vi "File Loader (SubVI).vi"(7 "Filename In":string) -> (0 "Number of Records":i32, 1 "Filename Out":string, 2 "output cluster":T1)   [LabVIEW 2014]
uses:
  <vilib>/Utility/file.llb/Read From Spreadsheet File (DBL).vi
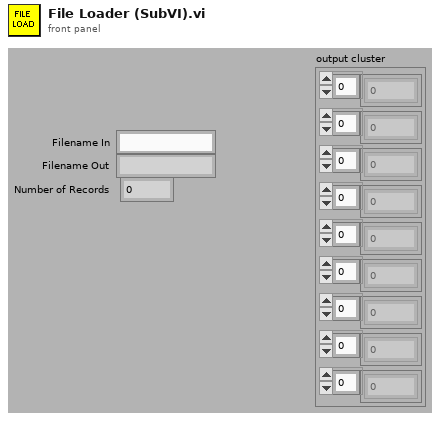
[diagram p1: front panel]
types:
  T1 = cluster{dbl[], dbl[], dbl[], dbl[], dbl[], dbl[], dbl[], dbl[], dbl[]}
  T2 = enum16{"open", "replace", "create", "open or create", "replace or create", "replace or create with confirmation"}
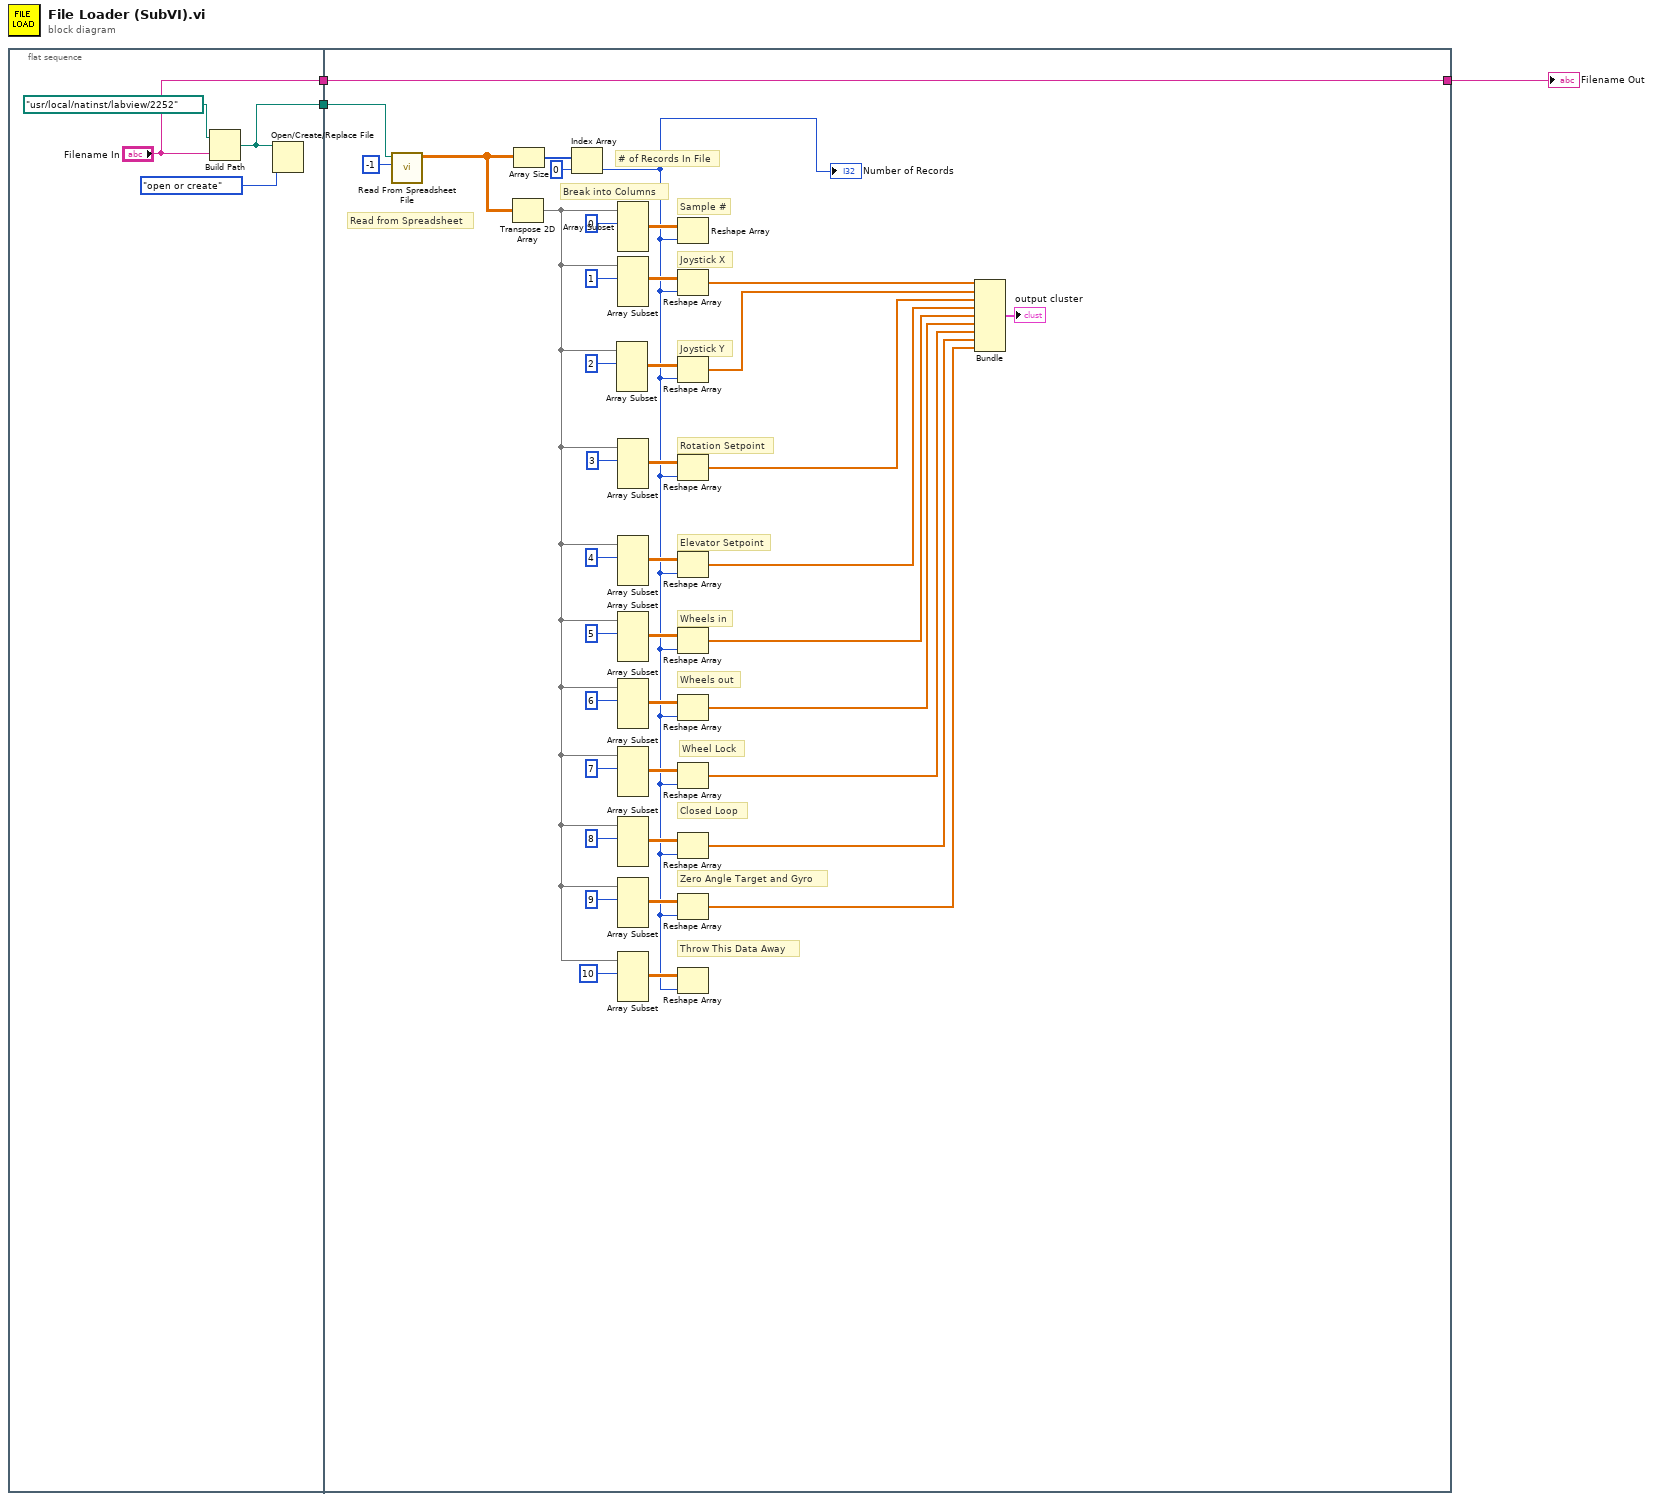
[diagram p0: block diagram]
diagram:
  n1 = flat-sequence {
    tunnel: [w6] -> w3
    tunnel: ["Filename In"] -> w1
    tunnel: w3 -> [w37]
    tunnel: [w34] -> w2
    tunnel: w1 -> [w34]
    frame #0 {
      n2 = Build Path(base path=path "/usr/local/natinst/labview/2252", name or relative path="Filename In") -> (appended path=w6:path)
      n3 = Open/Create/Replace File(file path (use dialog)=w6, operation (0:open)=T2."open or create") -> ()  [unwired: 1 in, 6 out]
    }
    frame #1 {
      # "Wheel Lock"
      # "Throw This Data Away"
      # "Zero Angle Target and Gyro"
      # "Closed Loop"
      # "Wheels out"
      # "Wheels in"
      # "Rotation Setpoint"
      # "Elevator Setpoint"
      # "Break into Columns"
      # "Read from Spreadsheet"
      # "# of Records In File"
      # "Joystick Y"
      # "Joystick X"
      # "Sample #"
      n4 = call-poly <vilib>:"Read From Spreadsheet File.vi"("number of rows (all:-1)"=-1, "file path (dialog if empty)"=w37) -> ("all rows"=w40:dbl[][])  [unwired: 2 in, 7 out]
      n5 = Transpose 2D Array(2D array=w40) -> (transposed array=w10:dbl[][])
      n6 = Array Size(array=w40) -> (size(s)=w39:i32[])
      n7 = Index Array(array=w39, index=0) -> (element=w11:i32)
      "Number of Records" <- w11
      n8 = Array Subset(array=w10, index (row)=2 ("index")) -> (w46:dbl[][])  [unwired: 3 in]
      n9 = Array Subset(array=w10, index (row)=0 ("index")) -> (w44:dbl[][])  [unwired: 3 in]
      n10 = Array Subset(array=w10, index (row)=1 ("index")) -> (w45:dbl[][])  [unwired: 3 in]
      n11 = Array Subset(array=w10, index (row)=3 ("index")) -> (w33:dbl[][])  [unwired: 3 in]
      n12 = Array Subset(array=w10, index (row)=4 ("index")) -> (w35:dbl[][])  [unwired: 3 in]
      n13 = Array Subset(array=w10, index (row)=5 ("index")) -> (w28:dbl[][])  [unwired: 3 in]
      n14 = Array Subset(array=w10, index (row)=6 ("index")) -> (w25:dbl[][])  [unwired: 3 in]
      n15 = Array Subset(array=w10, index (row)=7 ("index")) -> (w24:dbl[][])  [unwired: 3 in]
      n16 = Array Subset(array=w10, index (row)=8 ("index")) -> (w21:dbl[][])  [unwired: 3 in]
      n17 = Array Subset(array=w10, index (row)=9 ("index")) -> (w19:dbl[][])  [unwired: 3 in]
      n18 = Array Subset(array=w10, index (row)=10 ("index")) -> (w13:dbl[][])  [unwired: 3 in]
      n19 = Reshape Array(w44, w11) -> ()  [unwired: 1 out]
      n20 = Reshape Array(w45, w11) -> (w31:dbl[])
      n21 = Reshape Array(w46, w11) -> (w30:dbl[])
      n22 = Reshape Array(w33, w11) -> (w29:dbl[])
      n23 = Reshape Array(w35, w11) -> (w18:dbl[])
      n24 = Reshape Array(w28, w11) -> (w17:dbl[])
      n25 = Reshape Array(w25, w11) -> (w16:dbl[])
      n26 = Reshape Array(w24, w11) -> (w15:dbl[])
      n27 = Reshape Array(w21, w11) -> (w14:dbl[])
      n28 = Reshape Array(w19, w11) -> (w9:dbl[])
      n29 = Reshape Array(w13, w11) -> ()  [unwired: 1 out]
      n30 = Bundle(w31, w30, w29, w18, w17, w16, w15, w14, w9) -> (→"output cluster":T1)  [unwired: 1 in]
    }
  }
  "Filename Out" <- w2
